vi "Flatten Packet To Message String.vi"(8 "error in (no error)":errorcluster, 10 "Message Packet":variant, 11 "LogEventMessageProtocol in":refnum<class "LogEventMessageProtocol.lvclass">) -> (0 "error out":errorcluster, 3 "Packet as Message String":string)   [LabVIEW 2017, in "Network Sink.lvlib" / "LogEventMessageProtocol.lvclass"]
uses:
  <vilib>/gpm_packages/@cs/event-logger/Source/Network Sink/LogEventMessageProtocol/LogEventMessageProtocol.lvclass
  <vilib>/gpm_packages/@cs/event-logger/Source/Composed Log/Types/Log Packet.ctl
  <vilib>/gpm_packages/@cs/event-logger/Source/Composed Log/Types/Log Level.ctl
  <vilib>/gpm_packages/@cs/event-logger/Source/Composed Log/Composed Log.lvlib
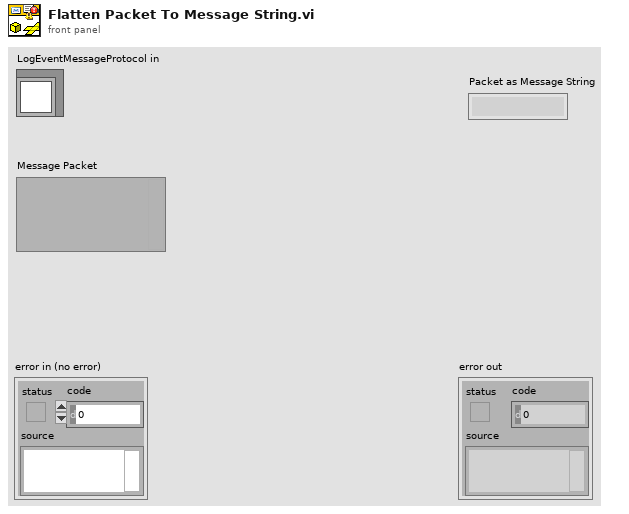
[diagram p1: front panel]
types:
  T1 = typedef "Composed Log.lvlib/Log Packet.ctl" = cluster{"Data To Log":string, "Source":string, "Event Level":T2, "Event Time":timestamp}
  T2 = typedef "Composed Log.lvlib/Log Level.ctl" = enum16{"Debug", "Info", "Warning", "Error", "Critical"}
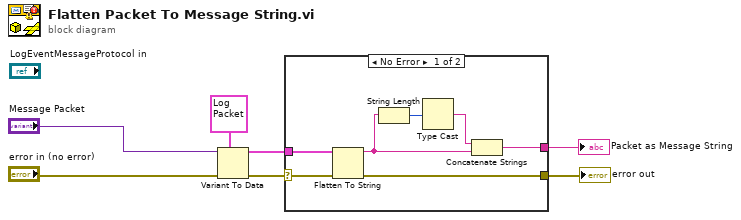
[diagram p0: block diagram]
diagram:
  n1 = Variant To Data(error in="error in (no error)", type=T1 {"Data To Log"="", "Source"="", "Event Level"=enum."Debug", "Event Time"=timestamp(0 s since 1904-01-01)} ("Log Packet"), Variant="Message Packet") -> (data=w3:T1, error out=w4:errorcluster)
  n2 = case shown="No Error" w4 {
    selector: w4 -> [w13 w15]
    tunnel: w3 -> [w14 _]
    tunnel: [w9 _] -> w2
    tunnel: [w8 w15] -> w1
    frame No Error {
      n3 = Flatten To String(anything=w14, error in (no error)=w13) -> (data string=w10:string, error out=w8:errorcluster)  [unwired: 2 in, 1 out]
      n4 = String Length(string=w10) -> (length=w12:i32)
      n5 = Type Cast(x=w12) -> (*(type *) &x=w11:string)  [unwired: 1 in]
      n6 = Concatenate Strings(w11, w10) -> (w9:string)
    }
    frame Error {
    }
  }
  "error out" <- w1
  "Packet as Message String" <- w2
